vi "tsa_AR Predict Error.vi"(0 "Xt":dbl[](array[numeric]) format="%.2f", 2 "AR coefficents":dbl[](array[numeric]) format="%.2f") -> (7 "error":dbl[](array[numeric]) format="%.10f", 10 "error":i32)   [LabVIEW 2018, in "NI_AALPro.lvlib"]
uses:
  NI_AALPro.lvlib
  IIR Filter (DBL).vi
  NI_AALBase.lvlib
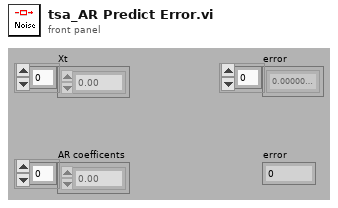
[diagram p1: front panel]
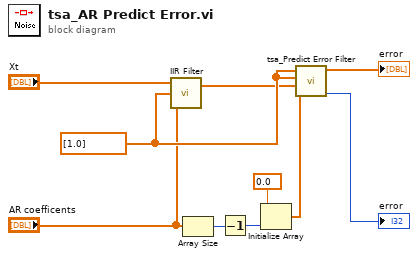
[diagram p0: block diagram]
diagram:
  w10 = dbl[] [1.0] ("Reverse Coefficients")
  n1 = call-poly "IIR Filter.vi"("Forward Coefficients"="AR coefficents", "Reverse Coefficients"=w10, "X"="Xt") -> ("Filtered X"=w2:dbl[])  [unwired: 1 in, 1 out]
  n2 = Array Size(array="AR coefficents") -> (size(s)=w8:i32)
  n3 = Decrement(x=w8) -> (x-1=w7:i32)
  n4 = Initialize Array(0.0 ("element"), w7) -> (w5:dbl[])
  n5 = call "tsa_Predict Error Filter.vi"("initial condition"=w5, "input signal"=w2, "A vector"=w10, "B vector"=w10) -> ("error"=→"error":i32, "output signal"=→"error":dbl[])  [unwired: 6 in]
